vi "Read Shared Library.vi"(8 "Error In":errorcluster, 11 "Session In":refnum<class "Session.lvclass">) -> (0 "Erorr Out":errorcluster, 2 "libssh2lv Shared Library":path, 3 "Session Out":refnum<class "Session.lvclass">)   [LabVIEW 2021, in "Field_RnD_Services_LIBSSH2_Toolkit.lvlib" / "Session.lvclass"]
doc: "Gets the path to the libssh2lv shared library used to interface with a remote SSH/SFTP server."
uses:
  220524-VNA RP FLAT.llb/Session.lvclass
  220524-VNA RP FLAT.llb/Session.lvclass/Session.ctl
  220524-VNA RP FLAT.llb/SSH.lvclass
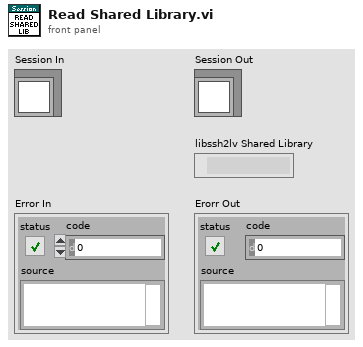
[diagram p1: front panel]
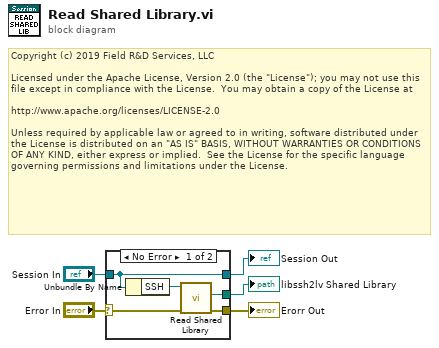
[diagram p0: block diagram]
diagram:
  # "Copyright (c) 2019 Field R&D Services, LLC\n\nLicensed under the Apache License, Version 2.0 (the \"License\"); you may not use this file except in compliance with the License.  You may obtain a copy of the License at\n\nhttp://www.apache.org/licenses/LICENSE-2.0\n\nUnless required by applicable law or agreed to in writing, software distributed under the License is distributed on an \"AS IS\" BASIS, WITHOUT WARRANTIES OR CONDITIONS OF ANY KIND, either express or implied.  See the License for the specific language governing permissions and limitations under the License."
  n1 = case shown="No Error" "Error In" {
    selector: "Error In" -> [w7 w11]
    tunnel: [w6 w11] -> w4
    tunnel: "Session In" -> [w10 w12]
    tunnel: [w10 w12] -> w2
    tunnel: [w8 _] -> w1
    frame No Error {
      n2 = Unbundle By Name(w10) -> ("SSH"=w9:refnum<class "SSH.lvclass">)
      n3 = call "Read Shared Library.vi"("Error In"=w7, "SSH In"=w9) -> ("Error Out"=w6:errorcluster, "libssh2lv Shared Library"=w8:path)  [unwired: 7 in, 1 out]
    }
    frame Error {
    }
  }
  "Erorr Out" <- w4
  "Session Out" <- w2
  "libssh2lv Shared Library" <- w1
